vi "Get Max and Min Flow Limits.vi"(2 "Current Step ID":i32, 3 "Tablle":string[][](array[string])) -> (0 "Max":dbl, 1 "Min":dbl)   [LabVIEW 2018]
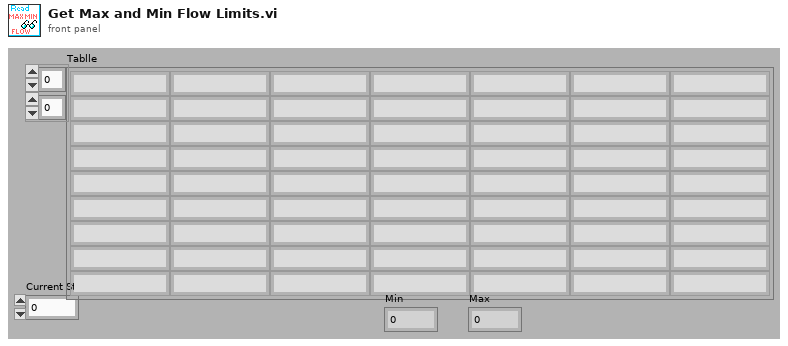
[diagram p1: front panel]
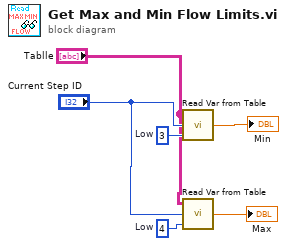
[diagram p0: block diagram]
diagram:
  w4 = 4  # Low
  w6 = 3  # Low
  n1 = call "Read Var from Table.vi"("VAR Column Index"=w6, "Current Step ID"="Current Step ID", "Value"="Tablle") -> ("Numeric"=→"Min":dbl)
  n2 = call "Read Var from Table.vi"("VAR Column Index"=w4, "Current Step ID"="Current Step ID", "Value"="Tablle") -> ("Numeric"=→"Max":dbl)
